vi "Read Fiducials.vi"(7 "Dispose Images?":bool=TRUE, 8 "error in":errorcluster, 9 "Fiducial Acquisition Parameters":T5, 10 "Location/Orientation in":T6, 11 "CameraTool in":refnum<class "CameraTool Class.lvclass">) -> (0 "error out":errorcluster, 2 "Fiducials":T1[](array[typedef]), 3 "CameraTool out":refnum<class "CameraTool Class.lvclass">)   [LabVIEW 2011, in "CameraTool Class.lvclass"]
uses:
  CameraTool Class.lvclass
  Utils/Type Definitions/Position_Orientation.ctl
  Vec3d Class/Vec3d Class.lvclass
  Orient3d Class/Orient3d Class.lvclass
  Utils/Type Definitions/Fiducial Image.ctl
  Utils/Type Definitions/Physical Image.ctl
  <vilib>/vision/Image Controls.llb/IMAQ Image.ctl
  Utils/Type Definitions/Fiducial with Source.ctl
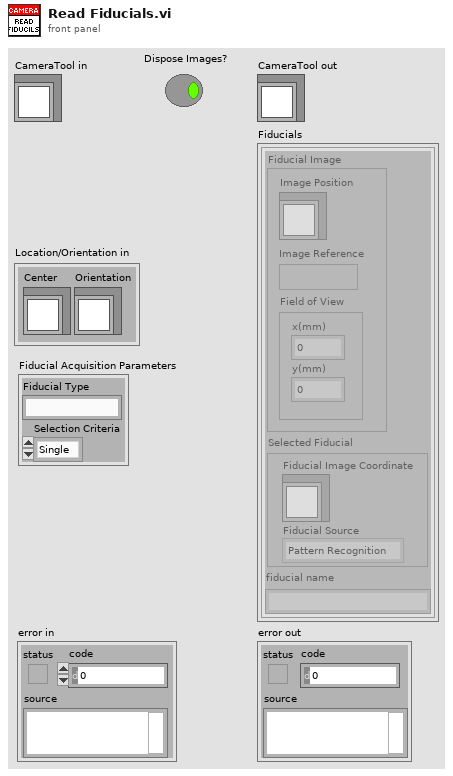
[diagram p1: front panel]
types:
  T1 = typedef "Fiducial Image.ctl" = cluster{"Fiducial Image":T2, "Selected Fiducial":T4, "fiducial name":string}
  T2 = typedef "Physical Image.ctl" = cluster{"Image Position":refnum<class "Vec3d Class.lvclass">, "Image Reference":T3, "Field of View":cluster{"x(mm)":dbl, "y(mm)":dbl}}
  T3 = typedef "IMAQ Image.ctl" = refnum<image>
  T4 = typedef "Fiducial with Source.ctl" = cluster{"Fiducial Image Coordinate":refnum<class "Vec3d Class.lvclass">, "Fiducial Source":enum16{"Pattern Recognition", "User", "Error", "Default"}}
  T5 = cluster{"Fiducial Type":string, "Selection Criteria":enum16{"Single", "Top", "Bottom"}}
  T6 = typedef "Position_Orientation.ctl" = cluster{"Center":refnum<class "Vec3d Class.lvclass">, "Orientation":refnum<class "Orient3d Class.lvclass">}
  T7 = cluster{"Feature Coordinates":refnum<class "Vec3d Class.lvclass">, "Feature Name":string}[]
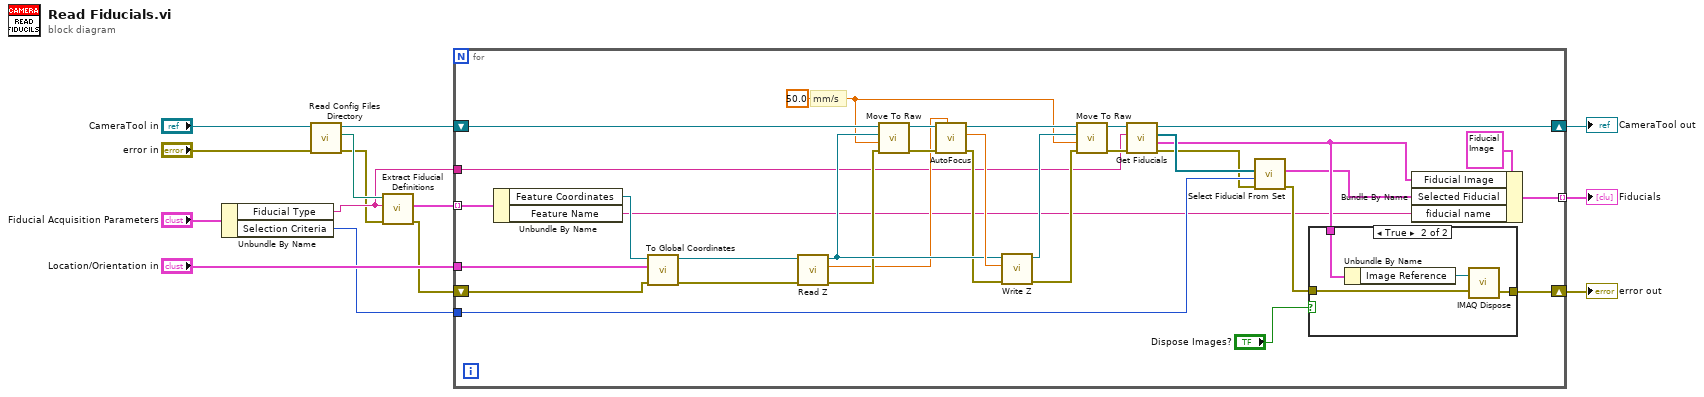
[diagram p0: block diagram]
diagram:
  n1 = Unbundle By Name("Fiducial Acquisition Parameters") -> ("Fiducial Type"=w5:string, "Selection Criteria"=w4:enum16{"Single", "Top", "Bottom"})
  n2 = call-dynamic "Read Config Files Directory.vi"("error in (no error)"="error in", "Gantry Class in"="CameraTool in") -> ("error out"=w1:errorcluster, "Config Files Directory"=w9:path, "Gantry Class out"=w11:refnum<class "CameraTool Class.lvclass">)  [unwired: 7 in]
  n3 = call "Extract Fiducial Definitions.vi"("error in"=w1, "Part Name"=w5, "Config Location"=w9) -> ("error out"=w7:errorcluster, "Feature Definitions"=w8:T7)  [unwired: 7 in]
  n4 = for {
    shift-right: [w25] -> w14
    shift-left: w11 -> [w47]
    shift-right: [w23] -> w3
    shift-left: w7 -> [w33]
    tunnel: "Location/Orientation in" -> [w36]
    tunnel: w8 -> [w35] mode=indexing
    tunnel: w5 -> [w28]
    tunnel: w4 -> [w26]
    tunnel: [w19] -> w2 mode=indexing
    w15 = 50.0
    # "mm/s"
    n5 = Unbundle By Name(w35) -> ("Feature Coordinates"=w34:refnum<class "Vec3d Class.lvclass">, "Feature Name"=w16:string)
    n6 = call "To Global Coordinates.vi"("error in"=w33, "Center/Orientation"=w36, "Local Coordinates"=w34) -> ("error out"=w37:errorcluster, "Global Coordinates"=w38:refnum<class "Vec3d Class.lvclass">)  [unwired: 7 in]
    n7 = call-dynamic "Read Z.vi"("error in (no error)"=w37, "Vec3d Class in"=w38) -> ("error out"=w41:errorcluster, "Z"=w30:dbl, "Vec3d Class out"=w44:refnum<class "Vec3d Class.lvclass">)  [unwired: 7 in]
    n8 = call-dynamic "Move To Raw.vi"("error in"=w41, "Speed"=w15, "Destination"=w44, "Gantry in"=w47) -> ("error out"=w46:errorcluster, "Gantry out"=w32:refnum<class "CameraTool Class.lvclass">)  [unwired: 6 in]
    n9 = call-dynamic "AutoFocus.vi"("Start Z"=w30, "error in"=w46, "CameraTool Class In"=w32) -> ("error out"=w40:errorcluster, "focus height"=w45:dbl, "CameraTool Class Out"=w31:refnum<class "CameraTool Class.lvclass">)  [unwired: 6 in]
    n10 = call-dynamic "Write Z.vi"("error in (no error)"=w40, "Z"=w45, "Vec3d Class in"=w44) -> ("error out"=w39:errorcluster, "Vec3d Class out"=w43:refnum<class "Vec3d Class.lvclass">)  [unwired: 7 in]
    n11 = call-dynamic "Move To Raw.vi"("error in"=w39, "Speed"=w15, "Destination"=w43, "Gantry in"=w31) -> ("error out"=w42:errorcluster, "Gantry out"=w29:refnum<class "CameraTool Class.lvclass">)  [unwired: 6 in]
    n12 = call "Get Fiducials.vi"("error in"=w42, "Fiducial Type"=w28, "CameraTool In"=w29) -> ("error out"=w24:errorcluster, "Fiducial Image"=w21:T2, "Fiducial Image Positions"=w27:refnum<class "Vec3d Class.lvclass">[], "CameraTool Out"=w25:refnum<class "CameraTool Class.lvclass">)  [unwired: 3 in]
    n13 = call "Select Fiducial From Set.vi"("error in"=w24, "Selection Criteria"=w26, "Fiducial Centers"=w27) -> ("error out"=w17:errorcluster, "Fiducial with Source"=w20:T4)  [unwired: 7 in]
    n14 = case shown="True" "Dispose Images?" {
      tunnel: [w48 w51] -> w23
      tunnel: w21 -> [_ w50]
      tunnel: w17 -> [w48 w49]
      frame False {
      }
      frame True {
        n15 = Unbundle By Name(w50) -> ("Image Reference"=w52:T3)
        n16 = call "IMAQ Dispose"("Image"=w52, "error in (no error)"=w49) -> ("error out"=w51:errorcluster)  [unwired: 4 in]
      }
    }
    n17 = Bundle By Name(cluster=T1 {"Fiducial Image"={"Image Position"=refnum, "Image Reference"=refnum, "Field of View"={"x(mm)"=0.0, "y(mm)"=0.0}}, "Selected Fiducial"={"Fiducial Image Coordinate"=refnum, "Fiducial Source"=enum."Pattern Recognition"}, "fiducial name"=""} ("Fiducial Image"), "Fiducial Image"=w21, "Selected Fiducial"=w20, "fiducial name"=w16) -> (w19:T1)
  }
  "error out" <- w3
  "CameraTool out" <- w14
  "Fiducials" <- w2
